vi "eye leveling.vi"(0 "Input array":u8[][](array[numeric]), 1 "Edge_offset_ratio":dbl, 2 "Intensity Thr":dbl, 3 "Image_Length":dbl, 4 "Top_cutoff":dbl) -> (5 "probe angle":cdb[](array[numeric]), 6 "scale":cdb[](array[numeric]))   [LabVIEW 2024]
uses:
  <vilib>/Math Plots/2D Math Plots/2D Compass/2D Compass XCtrl/2D Compass.xctl
  <vilib>/Math Plots/2D Math Plots/2D Compass/2D Compass Datatype/Public/Plot Helper (Complex).vi
  <vilib>/Math Plots/2D Math Plots/2D Compass/2D Compass Datatype/2D Compass Datatype.lvclass
  <vilib>/Math Plots/2D Math Plots/2D Plot/2D Plot Datatype/2D Plot Datatype.lvclass
panel:
  out "Original Graph":u8[][](graph)
  out "2D Compass":refnum<class "2D Plot Datatype.lvclass">[](xcontrol)
  out "Location2":dbl
  out "Location2":u8[][](graph)
  out "Location4":dbl
  out "Location4":u8[][](graph)
  out "Location3":dbl
  out "Location3":u8[][](graph)
  out "Location1":dbl
  out "Location1":u8[][](graph)
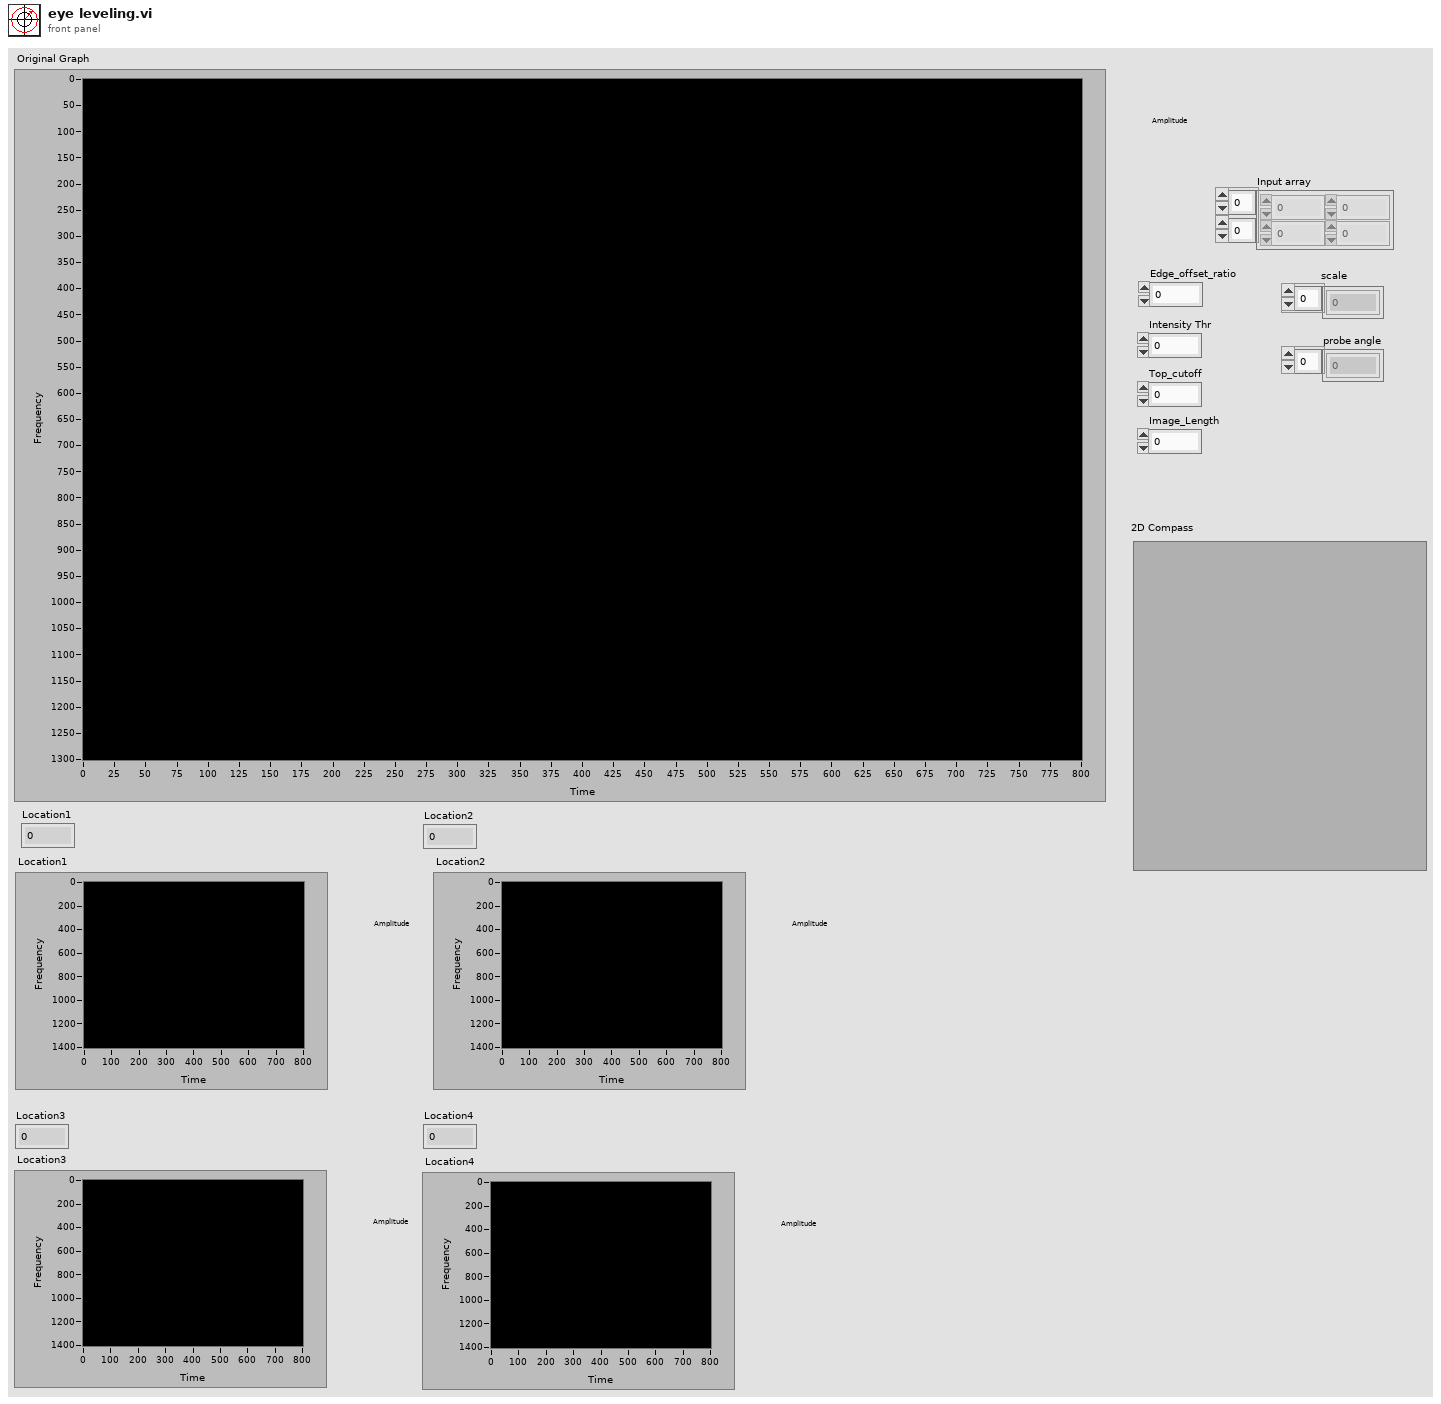
[diagram p1: front panel]
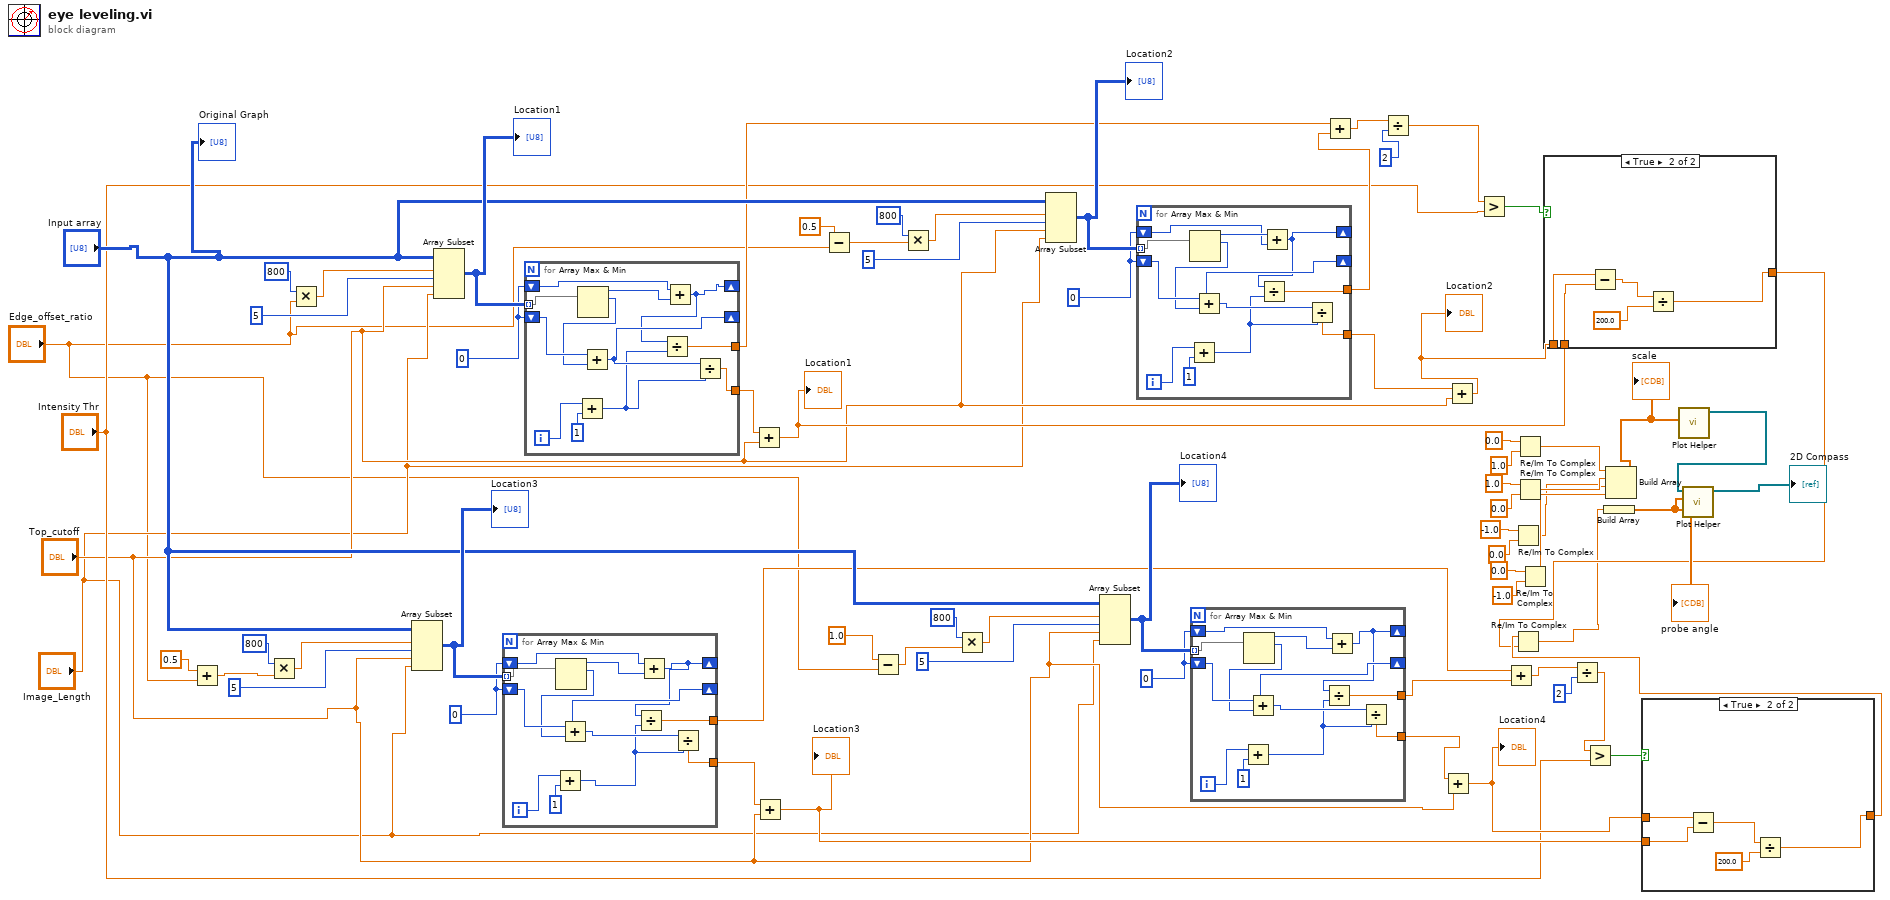
[diagram p0: block diagram]
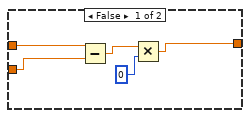
[diagram p2: hidden frame]
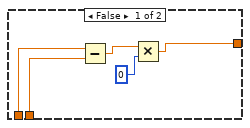
[diagram p3: hidden frame]
diagram:
  w13 = 0
  w12 = 0
  w14 = 0
  w15 = 0
  n1 = Add(x=0.5, y="Edge_offset_ratio") -> (x+y=w4:dbl)
  n2 = Multiply(x=800, y=w4) -> (x*y=w35:dbl)
  n3 = Multiply(x=800, y="Edge_offset_ratio") -> (x*y=w53:dbl)
  n4 = Array Subset(array="Input array", index (row)=w35, length (row)=5, index (col)="Top_cutoff", length (col)="Image_Length") -> (w65:u8[][])
  "Location3" <- w65
  n5 = Array Subset(array="Input array", index (row)=w53, length (row)=5, index (col)="Top_cutoff", length (col)="Image_Length") -> (w68:u8[][])
  "Location1" <- w68
  n6 = for {
    tunnel: w65 -> [w82] mode=indexing
    shift-right: [w77] -> _
    shift-left: w14 -> [w79]
    tunnel: [w81] -> w58
    shift-right: [w73] -> _
    shift-left: w14 -> [w74]
    tunnel: [w71] -> w24
    i -> [w76]
    n7 = Add(x=w76, y=1) -> (x+y=w72:i32)
    n8 = Array Max & Min(array=w82) -> (max value=w75:u8, max index (indices)=w78:i32)  [unwired: 2 out]
    n9 = Add(x=w79, y=w78) -> (x+y=w77:i32)
    n10 = Add(x=w74, y=w75) -> (x+y=w73:i32)
    n11 = Divide(x=w73, y=w72) -> (x/y=w71:dbl)
    n12 = Divide(x=w77, y=w72) -> (x/y=w81:dbl)
  }
  n13 = for {
    tunnel: w68 -> [w94] mode=indexing
    shift-right: [w89] -> _
    shift-left: w15 -> [w91]
    tunnel: [w93] -> w55
    shift-right: [w85] -> _
    shift-left: w15 -> [w86]
    tunnel: [w83] -> w32
    i -> [w88]
    n14 = Add(x=w88, y=1) -> (x+y=w84:i32)
    n15 = Array Max & Min(array=w94) -> (max value=w87:u8, max index (indices)=w90:i32)  [unwired: 2 out]
    n16 = Add(x=w91, y=w90) -> (x+y=w89:i32)
    n17 = Add(x=w86, y=w87) -> (x+y=w85:i32)
    n18 = Divide(x=w85, y=w84) -> (x/y=w83:dbl)
    n19 = Divide(x=w89, y=w84) -> (x/y=w93:dbl)
  }
  n20 = Add(x=w55, y="Top_cutoff") -> (x+y=w51:dbl)
  "Location1" <- w51
  n21 = Add(x=w58, y="Top_cutoff") -> (x+y=w25:dbl)
  "Location3" <- w25
  n22 = Subtract(x=0.5, y="Edge_offset_ratio") -> (x-y=w10:dbl)
  n23 = Subtract(x=1.0, y="Edge_offset_ratio") -> (x-y=w7:dbl)
  n24 = Multiply(x=800, y=w10) -> (x*y=w54:dbl)
  n25 = Multiply(x=800, y=w7) -> (x*y=w27:dbl)
  n26 = Array Subset(array="Input array", index (row)=w54, length (row)=5, index (col)="Top_cutoff", length (col)="Image_Length") -> (w59:u8[][])
  "Location2" <- w59
  n27 = Array Subset(array="Input array", index (row)=w27, length (row)=5, index (col)="Top_cutoff", length (col)="Image_Length") -> (w62:u8[][])
  "Location4" <- w62
  n28 = for {
    tunnel: w59 -> [w106] mode=indexing
    shift-right: [w101] -> _
    shift-left: w13 -> [w103]
    tunnel: [w105] -> w56
    shift-right: [w97] -> _
    shift-left: w13 -> [w98]
    tunnel: [w95] -> w31
    i -> [w100]
    n29 = Add(x=w100, y=1) -> (x+y=w96:i32)
    n30 = Array Max & Min(array=w106) -> (max value=w99:u8, max index (indices)=w102:i32)  [unwired: 2 out]
    n31 = Add(x=w103, y=w102) -> (x+y=w101:i32)
    n32 = Add(x=w99, y=w98) -> (x+y=w97:i32)
    n33 = Divide(x=w97, y=w96) -> (x/y=w95:dbl)
    n34 = Divide(x=w101, y=w96) -> (x/y=w105:dbl)
  }
  n35 = for {
    tunnel: w62 -> [w118] mode=indexing
    shift-right: [w113] -> _
    shift-left: w12 -> [w115]
    tunnel: [w117] -> w57
    shift-right: [w109] -> _
    shift-left: w12 -> [w110]
    tunnel: [w107] -> w23
    i -> [w112]
    n36 = Add(x=w112, y=1) -> (x+y=w108:i32)
    n37 = Array Max & Min(array=w118) -> (max value=w111:u8, max index (indices)=w114:i32)  [unwired: 2 out]
    n38 = Add(x=w115, y=w114) -> (x+y=w113:i32)
    n39 = Add(x=w110, y=w111) -> (x+y=w109:i32)
    n40 = Divide(x=w109, y=w108) -> (x/y=w107:dbl)
    n41 = Divide(x=w113, y=w108) -> (x/y=w117:dbl)
  }
  n42 = Add(x=w32, y=w31) -> (x+y=w30:dbl)
  n43 = Divide(x=w30, y=2) -> (x/y=w28:dbl)
  n44 = Add(x=w57, y="Top_cutoff") -> (x+y=w26:dbl)
  "Location4" <- w26
  n45 = Add(x=w56, y="Top_cutoff") -> (x+y=w52:dbl)
  "Location2" <- w52
  n46 = Greater?(x=w28, y="Intensity Thr") -> (0:w33:bool)
  n47 = Add(x=w24, y=w23) -> (x+y=w22:dbl)
  n48 = Re/Im To Complex(1:0.0 ("y"), 2:-1.0 ("x")) -> (0:w38:cdb)
  n49 = Re/Im To Complex(1:1.0 ("y"), 2:0.0 ("x")) -> (0:w40:cdb)
  n50 = Re/Im To Complex(1:0.0 ("y"), 2:1.0 ("x")) -> (0:w39:cdb)
  n51 = Re/Im To Complex(1:-1.0 ("y"), 2:0.0 ("x")) -> (0:w47:cdb)
  n52 = case shown="True" w33 {
    tunnel: w52 -> [w123 w128]
    tunnel: w51 -> [w122 w127]
    tunnel: [w119 w125] -> w2
    frame False {
      n53 = Subtract(x=w123, y=w122) -> (x-y=w121:dbl)
      n54 = Multiply(x=w121, y=0) -> (x*y=w119:dbl)
    }
    frame True {
      n55 = Subtract(x=w128, y=w127) -> (x-y=w126:dbl)
      n56 = Divide(x=w126, y=200.0) -> (x/y=w125:dbl)
    }
  }
  n57 = Divide(x=w22, y=2) -> (x/y=w20:dbl)
  n58 = Greater?(x=w20, y="Intensity Thr") -> (0:w18:bool)
  n59 = Build Array(w40, w39, w38, w47) -> (w36:cdb[])
  "scale" <- w36
  n60 = case shown="True" w18 {
    tunnel: [w131 w135] -> w3
    tunnel: w26 -> [w130 w138]
    tunnel: w25 -> [w129 w137]
    frame False {
      n61 = Subtract(x=w130, y=w129) -> (x-y=w133:dbl)
      n62 = Multiply(x=w133, y=0) -> (x*y=w131:dbl)
    }
    frame True {
      n63 = Subtract(x=w138, y=w137) -> (x-y=w136:dbl)
      n64 = Divide(x=w136, y=200.0) -> (x/y=w135:dbl)
    }
  }
  n65 = Re/Im To Complex(1:w2, 2:w3) -> (0:w1:cdb)
  n66 = Build Array(w1) -> (w11:cdb[])
  "probe angle" <- w11
  n67 = call-poly <vilib>:"Plot Helper.vi"("z vector"=w36) -> ("2D Plot Class Obj Array out"=w37:refnum<class "2D Plot Datatype.lvclass">[])  [unwired: 2 in, 8 out]
  n68 = call-poly <vilib>:"Plot Helper.vi"("z vector"=w11, "2D Plot Class Obj Array in"=w37) -> ("2D Plot Class Obj Array out"=→"2D Compass":refnum<class "2D Plot Datatype.lvclass">[])  [unwired: 1 in, 8 out]
  "Original Graph" <- "Input array"
